vi "Write Log file.vi"(10 "Log file":path, 11 "SolutionBuilder in":refnum<class "SolutionBuilder.lvclass">) -> (3 "SolutionBuilder out":refnum<class "SolutionBuilder.lvclass">)   [LabVIEW 2019, in "SolutionBuilder.lvlib" / "SolutionBuilder.lvclass"]
uses:
  SolutionBuilder.lvclass
  SolutionBuilder.lvclass/SolutionBuilder.ctl
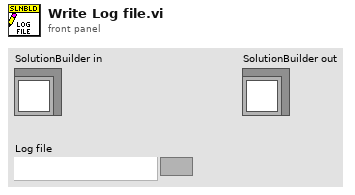
[diagram p1: front panel]
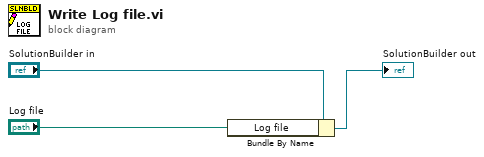
[diagram p0: block diagram]
diagram:
  n1 = Bundle By Name(cluster="SolutionBuilder in", "Log file"="Log file") -> (→"SolutionBuilder out":refnum<class "SolutionBuilder.lvclass">)
